vi "DPO_7K_Set_Edge_Trigger.vi"(5 "Trigger Slope":u16(ring) items=["Rising", "Falling", "Either"], 6 "Trigger Level":dbl, 7 "Trigger Coupling":u16(ring) items=["AC", "DC", "HF Reject (>50 kHz)", "LF Reject (<80 kHz)", "Noise Reject"], 8 "Error In":errorcluster, 9 "Trigger Channel":u16(ring) items=["Channel 1", "Channel 2", "Channel 3", "Channel 4", "Auxiliary", "Line"], 10 "Trigger Mode":u16(ring) items=["Auto", "Normal"], 11 "VISA resource name in":refnum<visa-resource-name>) -> (0 "Error Out":errorcluster, 3 "VISA resource name out":refnum<visa-resource-name>)   [LabVIEW 2020]
uses:
  subVI/Return_To_Interface.ctl
  subVI/Set_Configuration.ctl
panel:
  in  "Set":T1
  in  "Return to Interface":T2
  # "SET TRIGGER MODE"
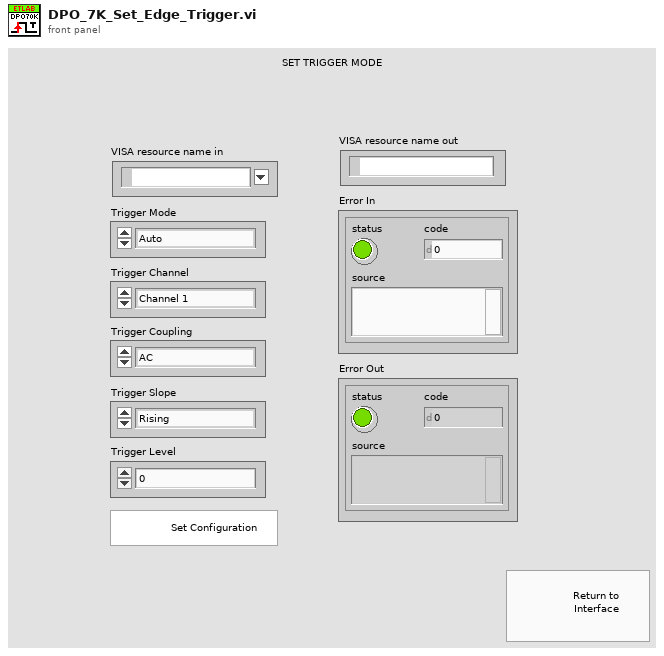
[diagram p1: front panel]
types:
  T1 = typedef "Set_Configuration.ctl" = bool
  T2 = typedef "Return_To_Interface.ctl" = bool
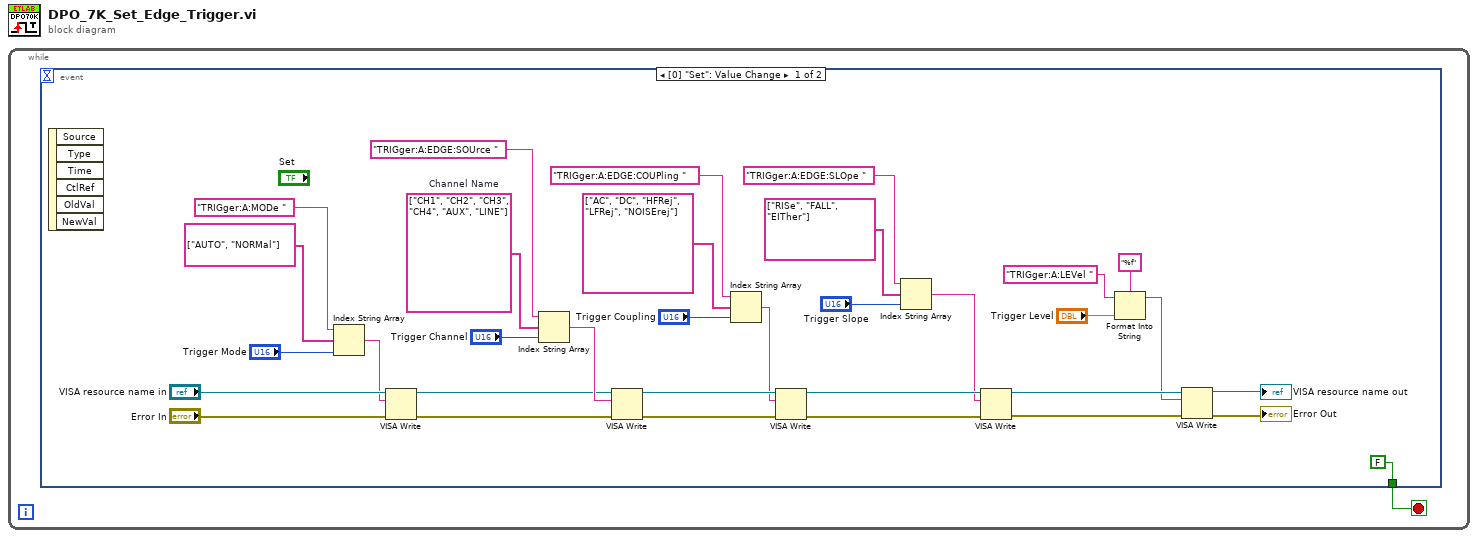
[diagram p0: block diagram]
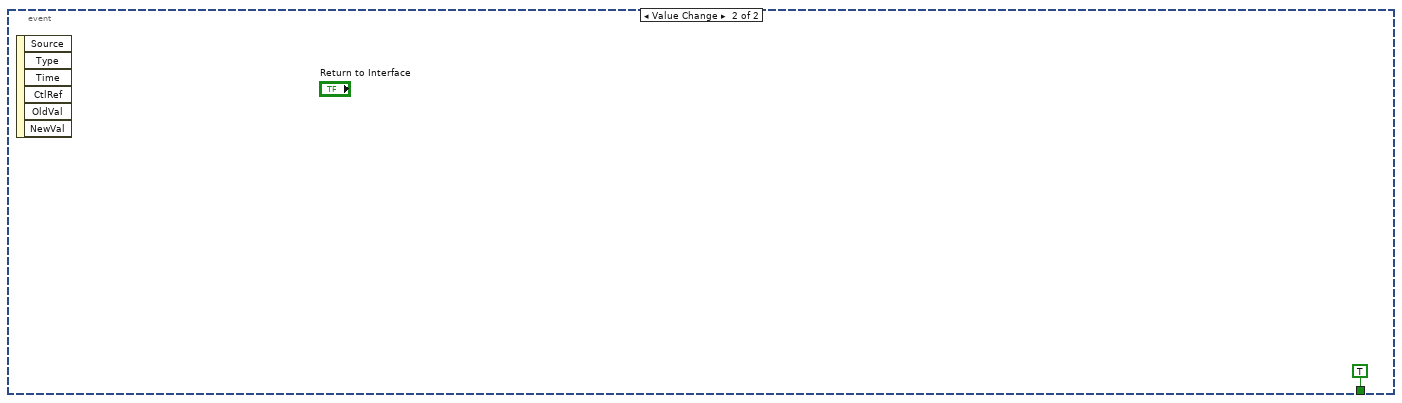
[diagram p2: hidden frame]
diagram:
  n1 = while {
    stop <- w1 stop-if-true
    n2 = event shown="[0] \"Set\": Value Change" {
      selector: _ -> [_ _]
      dyn-events: _ -> [_ _]
      timeout: _ -> [_ _]
      tunnel: [FALSE TRUE] -> w1
      event Value Change {
        w34 = string[] ["CH1", "CH2", "CH3", "CH4", "AUX", "LINE"]  # Channel Name
        n3 = event-data() -> ()  [unwired: 1 in, 6 out]
        n4 = Index String Array(1:"Trigger Mode", 2:string[] ["AUTO", "NORMal"], 3:"TRIGger:A:MODe ") -> (0:w11:string)
        n5 = VISA Write(VISA resource name="VISA resource name in", write buffer=w11, error in (no error)="Error In") -> (VISA resource name out=w13:refnum<visa-resource-name>, error out=w12:errorcluster)  [unwired: 1 out]
        n6 = Index String Array(1:"Trigger Channel", 2:w34, 3:"TRIGger:A:EDGE:SOUrce ") -> (0:w23:string)
        n7 = VISA Write(VISA resource name=w13, write buffer=w23, error in (no error)=w12) -> (VISA resource name out=w32:refnum<visa-resource-name>, error out=w31:errorcluster)  [unwired: 1 out]
        n8 = Index String Array(1:"Trigger Coupling", 2:string[] ["AC", "DC", "HFRej", "LFRej", "NOISErej"], 3:"TRIGger:A:EDGE:COUPling ") -> (0:w25:string)
        n9 = VISA Write(VISA resource name=w32, write buffer=w25, error in (no error)=w31) -> (VISA resource name out=w21:refnum<visa-resource-name>, error out=w20:errorcluster)  [unwired: 1 out]
        n10 = Index String Array(1:"Trigger Slope", 2:string[] ["RISe", "FALL", "EITher"], 3:"TRIGger:A:EDGE:SLOpe ") -> (0:w19:string)
        n11 = VISA Write(VISA resource name=w21, write buffer=w19, error in (no error)=w20) -> (VISA resource name out=w10:refnum<visa-resource-name>, error out=w9:errorcluster)  [unwired: 1 out]
        n12 = Format Into String(format string="%f", initial string="TRIGger:A:LEVel " ("format string"), "Trigger Level") -> (resulting string=w4:string)  [unwired: 1 in, 1 out]
        n13 = VISA Write(VISA resource name=w10, write buffer=w4, error in (no error)=w9) -> (VISA resource name out=→"VISA resource name out":refnum<visa-resource-name>, error out=→"Error Out":errorcluster)  [unwired: 1 out]
      }
      event Value Change {
        n14 = event-data() -> ()  [unwired: 1 in, 6 out]
      }
    }
  }
